vi "EMC_Stop_Contour.vi"(8 "error in (no error)":errorcluster, 11 "coordinate":refnum<k21>) -> (0 "error out":errorcluster)   [LabVIEW 2015]
uses:
  EMC_Typedef_Motor_Parameters.ctl
  <vilib>/Motion/PropertyNodes/nimc.createStopMoveInstance.coordinate.vi
  <vilib>/Motion/PropertyNodes/nimc.destroyInterfaceInstance.vi
  <resource>/objmgr/nimotion.rc
panel:
  in  "table":refnum<k21>
  in  "Motion Parameters":T1={"position"=1000.0, "velocity"=1000.0, "acceleration"=10000.0, "deceleration"=10000.0, "accel. jerk"=10000.0, "decel. jerk"=10000.0}
  in  "axis":refnum<k21>
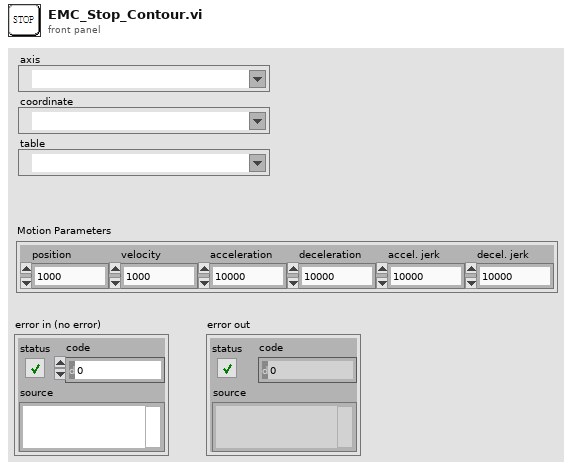
[diagram p1: front panel]
types:
  T1 = typedef "EMC_Typedef_Motor_Parameters.ctl" = cluster{"position":dbl, "velocity":dbl, "acceleration":dbl, "deceleration":dbl, "accel. jerk":dbl, "decel. jerk":dbl}
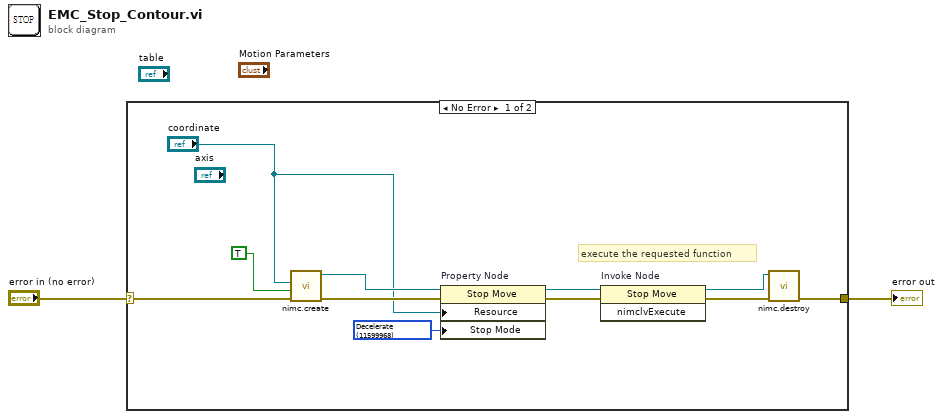
[diagram p0: block diagram]
diagram:
  n1 = case shown="No Error" "error in (no error)" {
    selector: "error in (no error)" -> [w5 w14]
    tunnel: [w8 w14] -> w2
    frame No Error {
      w4 = 11599968 items=["Decelerate"=11599968, "Immediate"=11599969, "Disable Drive"=11599970] ("Stop Mode")
      # "execute the requested function"
      n2 = call-poly <vilib>:"nimc.create.vi"("error in"=w5, "async?"=TRUE ("execute asynchronously?"), "coordinate"="coordinate") -> ("error out"=w11:errorcluster, "stop"=w6:refnum<k20>)  [unwired: 6 in, 1 out]
      n3 = property on="Property Node" class="Stop Move"(reference=w6, error in=w11, "Resource"="coordinate", "Stop Mode"=w4) -> (reference out=w13:refnum<k20>, error out=w12:errorcluster)
      n4 = invoke on="Invoke Node" class="Stop Move" method="nimclvExecute"(reference=w13, error in=w12) -> (reference out=w10:refnum<k20>, error out=w9:errorcluster)  [unwired: 1 in, 1 out]
      n5 = call-poly <vilib>:"nimc.destroy.vi"("error in"=w9, "motion handle"=w10) -> ("error out"=w8:errorcluster)  [unwired: 9 in]
    }
    frame Error {
    }
  }
  "error out" <- w2
